vi "InputAudio.vi"(9 "Channel":dbl, 10 "path":path, 11 "Sample value":dbl) -> (1 "Centroid":dbl, 2 "data":waveform(dbl)[](array[waveform]), 3 "RMS":dbl, 4 "Roll up":dbl, 5 "BPM":dbl, 6 "Zero Crossing":dbl, 7 "Waveform Graph":waveform(dbl)[](graph))   [LabVIEW 2020]
uses:
  <vilib>/Analysis/5stat.llb/RMS (DBL).vi
  <vilib>/measure/mascope.llb/Amplitude and Levels N chan.vi
  <vilib>/Analysis/NI_AALPro.lvlib
  <vilib>/measure/NI_MAPro.lvlib
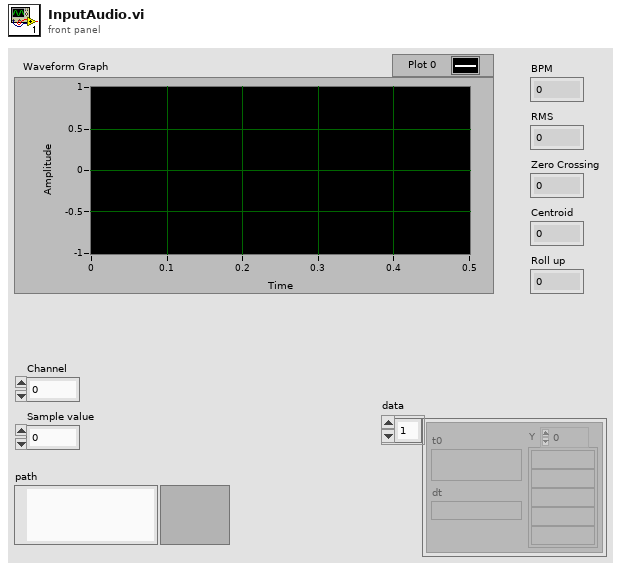
[diagram p1: front panel]
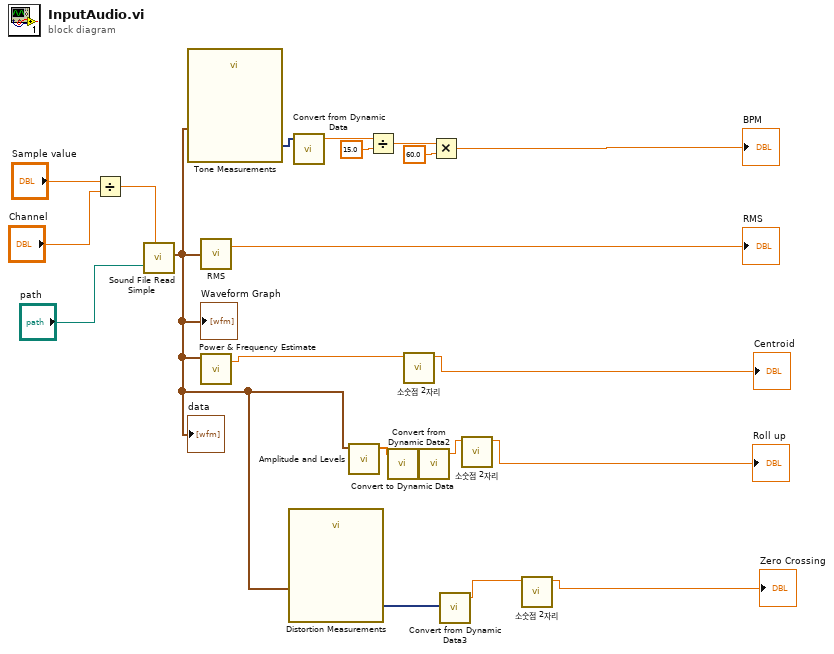
[diagram p0: block diagram]
diagram:
  n1 = Divide(x="Sample value", y="Channel") -> (x/y=w5:dbl)
  n2 = call <vilib>:"Sound File Read Simple.vi"("number of samples/ch (-1: all)"=w5, "path"="path") -> ("data"=w14:waveform(dbl)[])  [unwired: 6 in, 3 out]
  "Waveform Graph" <- w14
  "data" <- w14
  n3 = call "Tone Measurements"("Signals"=w14) -> ("Frequency"=w6:dynamicdata)  [unwired: 9 in, 1 out]
  n4 = call-poly <vilib>:"RMS.vi"("X"=w14) -> ("rms value"=→"RMS":dbl)  [unwired: 1 out]
  n5 = call <vilib>:"Power & Frequency Estimate.vi"("Power Spectrum (V^2 rms)"=w14) -> ("est frequency peak"=w16:dbl)  [unwired: 5 in, 1 out]
  n6 = call "Distortion Measurements"("Signals"=w14) -> ("SINAD (dB)"=w15:dynamicdata)  [unwired: 9 in, 1 out]
  n7 = call "Convert from Dynamic Data"("Dynamic Data Type"=w6) -> ("Scalar"=w7:dbl)  [unwired: 3 in]
  n8 = call-poly <vilib>:"Amplitude and Levels.vi"("signal(s) in"=w14) -> ("amplitude"=w12:dbl[])  [unwired: 7 in, 3 out]
  n9 = Divide(x=w7, y=15.0) -> (x/y=w9:dbl)
  n10 = call "Convert to Dynamic Data"("Array"=w12) -> ("Dynamic Data Type"=w13:dynamicdata)  [unwired: 3 in]
  n11 = call "소숫점 2자리.vi"("input Value"=w16) -> ("output value"=→"Centroid":dbl)  [unwired: 10 in]
  n12 = call "Convert from Dynamic Data2"("Dynamic Data Type"=w13) -> ("Scalar"=w18:dbl)  [unwired: 3 in]
  n13 = Multiply(x=w9, y=60.0) -> (x*y=→"BPM":dbl)
  n14 = call "Convert from Dynamic Data3"("Dynamic Data Type"=w15) -> ("Scalar"=w20:dbl)  [unwired: 3 in]
  n15 = call "소숫점 2자리.vi"("input Value"=w18) -> ("output value"=→"Roll up":dbl)  [unwired: 10 in]
  n16 = call "소숫점 2자리.vi"("input Value"=w20) -> ("output value"=→"Zero Crossing":dbl)  [unwired: 10 in]
